vi "_wpt_subvi.vi"() -> ()   [LabVIEW 2019]
uses:
  Ctrl/waypoint_buf.ctl
panel:
  out "incircle waypts":cluster{"x":dbl, "y":dbl}[](array[cluster]) {"x" format="%.2f"; "y" format="%.2f"}
  out "waypoint analysis":T1
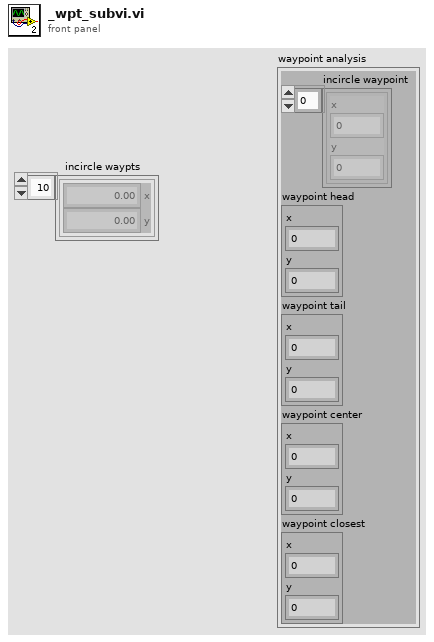
[diagram p1: front panel]
types:
  T1 = cluster{"incircle waypoint":cluster{"x":dbl, "y":dbl}[], "waypoint head":cluster{"x":dbl, "y":dbl}, "waypoint tail":cluster{"x":dbl, "y":dbl}, "waypoint center":cluster{"x":dbl, "y":dbl}, "waypoint closest":cluster{"x":dbl, "y":dbl}}
  T2 = typedef "waypoint_buf.ctl" = enum16{"clear", "write", "read"}
  T3 = cluster{"lookahead pt n":dbl, "lookahead distance":dbl}
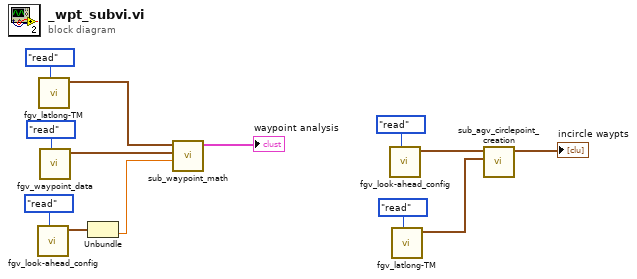
[diagram p0: block diagram]
diagram:
  n1 = call "fgv_look-ahead_config.vi"("cmd"=enum16{"read", "write"}."read") -> ("lookahed cfg out"=w10:T3)  [unwired: 10 in]
  n2 = call "fgv_latlong-TM.vi"("cmd"=enum16{"write", "read"}."read") -> ("tm out"=w7:cluster{dbl, dbl})  [unwired: 9 in, 1 out]
  n3 = call "fgv_waypoint_data.vi"("cmd"=waypoint_buf."read") -> ("waypoint out"=w12:cluster{"x":dbl, "y":dbl}[])  [unwired: 8 in, 2 out]
  n4 = Unbundle(w10) -> ("lookahead distance"=w8:dbl)  [unwired: 1 out]
  n5 = call "sub_waypoint_math.vi"("lookahead distance"=w8, "waypoint out"=w12, "tm out"=w7) -> ("waypoint analysis format"=→"waypoint analysis":T1)  [unwired: 8 in]
  n6 = call "fgv_look-ahead_config.vi"("cmd"=enum16{"read", "write"}."read") -> ("lookahed cfg out"=w5:T3)  [unwired: 10 in]
  n7 = call "fgv_latlong-TM.vi"("cmd"=enum16{"write", "read"}."read") -> ("tm out"=w2:cluster{dbl, dbl})  [unwired: 9 in, 1 out]
  n8 = call "sub_agv_circlepoint_creation.vi"("tm out"=w2, "lookahed cfg out"=w5) -> ("incircle waypoints"=→"incircle waypts":cluster{dbl, dbl}[])  [unwired: 9 in]
